vi "LineColorEnd.vi"(6 "Row":i32, 7 "Cluster":T1, 8 "error in":errorcluster, 9 "Event":bool, 11 "Result\n0.Item\n1.data\n2.limit\n3.result":string[](array[string])) -> (1 "SystemProcess":T2, 3 "Row":i32, 5 "output cluster":T1)   [LabVIEW 2013]
uses:
  Control/SystemProcess.ctl
  <vilib>/Utility/miscctls.llb/LVRowAndColumnTypeDef.ctl
  <vilib>/Utility/miscctls.llb/LVRowAndColumnUnsignedTypeDef.ctl
  Control/Read&Write.ctl
  Control/Buffer.vi
panel:
  out "Reserve:":string
  out "last":i32
  out "this":u32
  out "concatenated string":string
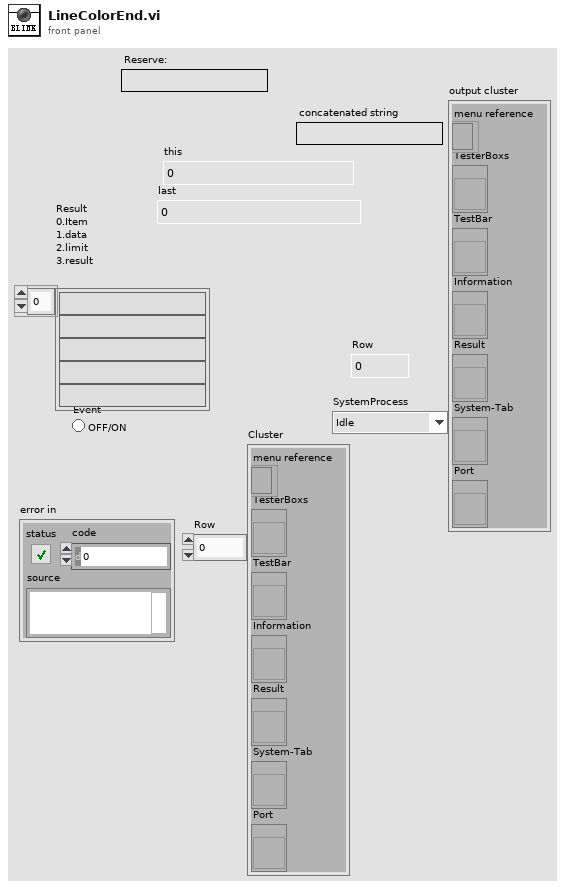
[diagram p1: front panel]
types:
  T1 = cluster{"menu reference":refnum<k9>, "TesterBoxs":refnum<vi>, "TestBar":refnum<vi>, "Information":refnum<vi>, "Result":refnum<vi>, "System-Tab":refnum<vi>, "Port":refnum<vi>}
  T2 = typedef "SystemProcess.ctl" = enum16{"Idle", "SystemInit", "SpecialEvent", "Barcode(SN)", "TestInitialize", "Test", "Stop", "SaveTestData", "Exit"}
  T3 = typedef "LVRowAndColumnUnsignedTypeDef.ctl" = cluster{"Row":u32, "Column":u32}
  T4 = typedef "LVRowAndColumnTypeDef.ctl" = cluster{"Row":i32, "Column":i32}
  T5 = typedef "Read&Write.ctl" = enum16{"Read", "Write"}
  T6 = typedef "StatusInformation.ctl" = cluster{"FileName:":string, "Barcode(S/N):":string, "TestStep:":string, "TestTime:":string, "Station:":string, "Model:":string, "Line:":string, "Status:":string, "Series:":string, "Reserve:":string}
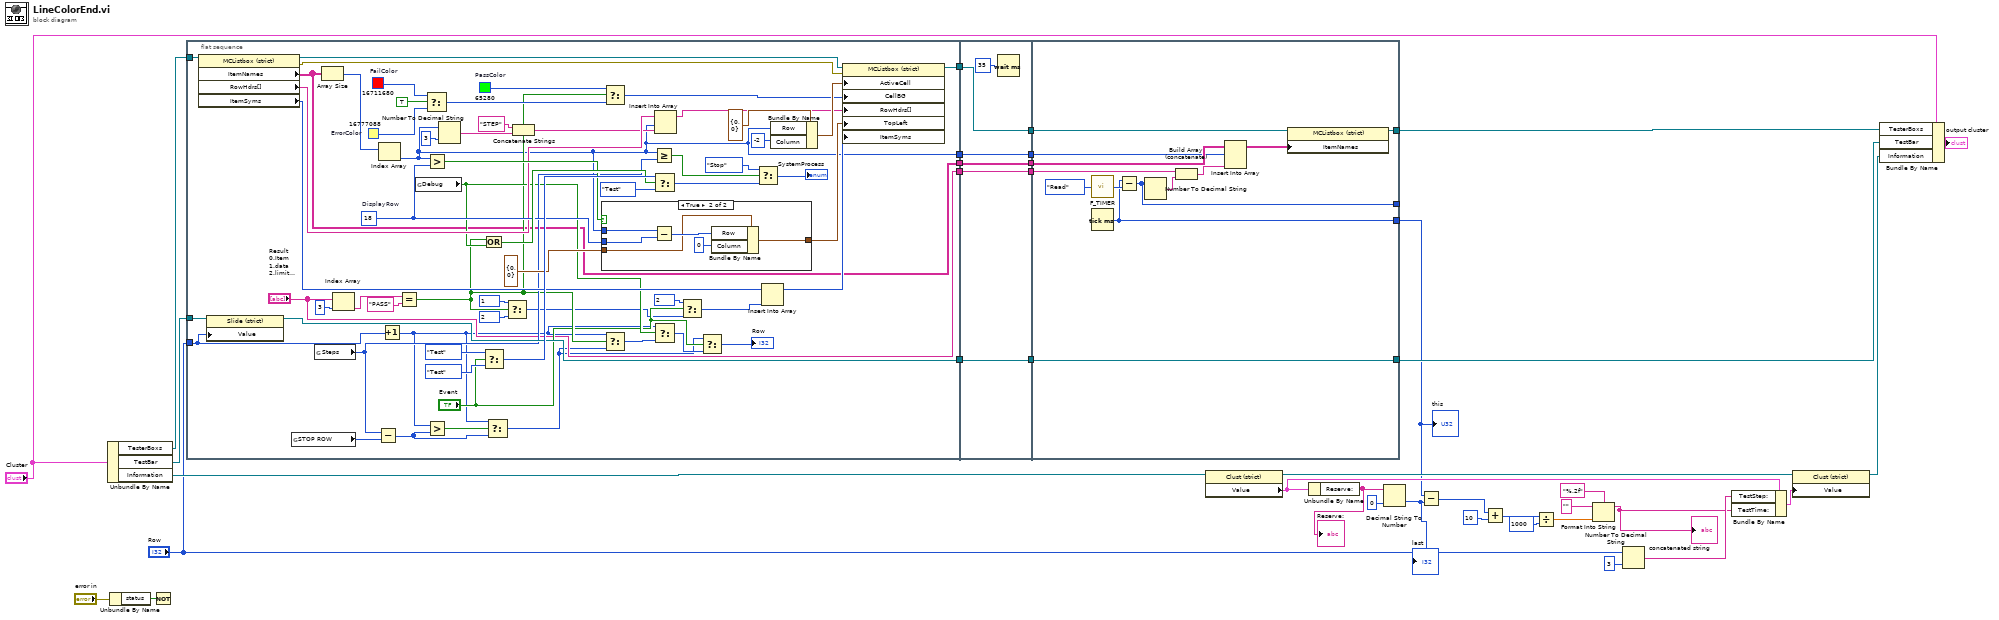
[diagram p0: block diagram]
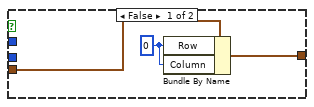
[diagram p2: hidden frame]
diagram:
  n1 = Unbundle By Name("Cluster") -> ("TesterBoxs"=w36:refnum<vi>, "TestBar"=w34:refnum<vi>, "Information"=w32:refnum<vi>)
  n2 = Unbundle By Name("error in") -> ("status"=w37:bool)
  n3 = Not(x=w37) -> ()  [unwired: 1 out]
  n4 = flat-sequence {
    tunnel: w36 -> [w67]
    tunnel: w34 -> [w65]
    tunnel: "Row" -> [w42]
    tunnel: [w66] -> w17
    tunnel: [w64] -> w15
    tunnel: [w46] -> w13
    tunnel: [w45] -> w11
    tunnel: ["Result\n0.Item\n1.data\n2.limit\n3.result"] -> w9
    tunnel: w17 -> [w114]
    tunnel: [w114] -> w16
    tunnel: w15 -> [w113]
    tunnel: [w113] -> w14
    tunnel: w13 -> [w112]
    tunnel: [w112] -> w12
    tunnel: w11 -> [w111]
    tunnel: [w111] -> w10
    tunnel: w9 -> [w110]
    tunnel: [w110] -> w8
    tunnel: [w127] -> w33
    tunnel: [w125] -> w35
    tunnel: [w116] -> w5
    tunnel: w8 -> [w119]
    tunnel: w10 -> [w122]
    tunnel: w12 -> [w123]
    tunnel: w14 -> [w127]
    tunnel: w16 -> [w126]
    tunnel: [w115] -> _
    frame #0 {
      w77 = 18  # DisplayRow
      w81 = u32 16777088  # ErrorColor
      w83 = u32 16711680  # FailColor
      w88 = u32 65280  # PassColor
      n5 = property class="MCListbox (strict)"(reference=w67) -> (reference out=w86:refnum<vi>, error out=w85:errorcluster, "ItemNames"=w46:string[][], "RowHdrs[]"=w73:string[], "ItemSyms"=w63:i32[])  [unwired: 1 in]
      n6 = property class="Slide (strict)"(reference=w65, "Value"=w42) -> (reference out=w64:refnum<vi>)  [unwired: 1 in, 1 out]
      n7 = global read "Buffer.vi" "STOP ROW"() -> (w47:i32)
      n8 = global read "Buffer.vi" "Steps"() -> (w59:i32)
      n9 = Array Size(array=w46) -> (size(s)=w84:i32[])
      n10 = Index Array(array="Result\n0.Item\n1.data\n2.limit\n3.result", index=3) -> (element=w93:string)
      n11 = Subtract(x=w59, y=w47) -> (x-y=w41:i32)
      n12 = Index Array(array=w84) -> (element=w45:i32)  [unwired: 1 in]
      n13 = Increment(x=w42) -> (x+1=w39:i32)
      n14 = Equal?(x=w93, y="PASS") -> (x = y?=w54:bool)
      n15 = global read "Buffer.vi" "Debug"() -> (w58:bool)
      n16 = Select(t=w83, s=TRUE, f=w81) -> (s? t:f=w82:u32)
      n17 = Greater?(x=w45, y=w77) -> (0:w78:bool)
      n18 = Greater?(x=w39, y=w41) -> (0:w43:bool)
      n19 = Number To Decimal String(number=w45, width (-)=i16 3) -> (decimal integer string=w69:string)
      n20 = Or(x=w54, y=w58) -> (x .or. y?=w80:bool)
      n21 = Select(t=SystemProcess."Test", s="Event", f=SystemProcess."Test") -> (s? t:f=w96:T2)
      n22 = Select(t=w39, s=w43, f=w41) -> (s? t:f=w40:i32)
      n23 = Select(t=1, s=w54, f=2) -> (s? t:f=w49:i32)
      n24 = Concatenate Strings("STEP" ("string"), w69) -> (w70:string)
      n25 = case shown="True" w78 {
        tunnel: w45 -> [_ w107]
        tunnel: [w102 w105] -> w75
        tunnel: w77 -> [_ w104]
        tunnel: T3 {"Row"=0, "Column"=0} ("Top Left Visible Cell") -> [w100 w103]
        frame False {
          w101 = u32 0 ("Column")
          n26 = Bundle By Name(cluster=w100, "Row"=w101, "Column"=w101) -> (w102:T3)
        }
        frame True {
          n27 = Subtract(x=w107, y=w104) -> (x-y=w106:i32)
          n28 = Bundle By Name(cluster=w103, "Row"=w106, "Column"=u32 0) -> (w105:T3)
        }
      }
      n29 = Select(t=w88, s=w54, f=w82) -> (s? t:f=w87:u32)
      n30 = Select(t=w39, s=w54, f=w40) -> (s? t:f=w57:i32)
      n31 = Greater Or Equal?(x=w45, y=w59) -> (x >= y?=w95:bool)
      n32 = Select(t=w96, s=w80, f=SystemProcess."Test") -> (s? t:f=w56:T2)
      n33 = Select(t=w39, s=w58, f=w57) -> (s? t:f=w53:i32)
      n34 = Insert Into Array(array=w73, index=w45, new element=w70) -> (w72:string[])
      n35 = Select(t=2, s="Event", f=w49) -> (s? t:f=w48:i32)
      n36 = Select(t=w40, s="Event", f=w53) -> (s? t:f=→"Row":i32)
      n37 = Select(t=SystemProcess."Stop" ("SystemProcess"), s=w95, f=w56) -> (s? t:f=→"SystemProcess":T2)
      n38 = Insert Into Array(array=w63, new element=w48) -> (w60:i32[])  [unwired: 1 in]
      n39 = Bundle By Name(cluster=T4 {"Row"=0, "Column"=0} ("Active Cell:Active Cell"), "Row"=w45, "Column"=-2) -> (w89:T4)
      n40 = property on="Property Node" class="MCListbox (strict)"(reference=w86, error in=w85, "ActiveCell"=w89, "CellBG"=w87, "RowHdrs[]"=w72, "TopLeft"=w75, "ItemSyms"=w60) -> (reference out=w66:refnum<vi>)  [unwired: 1 out]
    }
    frame #1 {
      n41 = Wait (ms)(milliseconds to wait=u32 35) -> ()  [unwired: 1 out]
    }
    frame #2 {
      n42 = call "F_TIMER.vi"("Enum-Read/Write"=Read&Write."Read") -> ("timer"=w121:u32)
      n43 = Tick Count (ms)() -> (millisecond timer value=w116:u32)
      n44 = Subtract(x=w116, y=w121) -> (x-y=w115:u32)
      n45 = Number To Decimal String(number=w115) -> (decimal integer string=w118:string)  [unwired: 1 in]
      n46 = Build Array (concatenate)(w119, w118) -> (w117:string[])
      n47 = Insert Into Array(array=w123, index (row)=w122, new element=w117) -> (w124:string[][])  [unwired: 1 in]
      n48 = property class="MCListbox (strict)"(reference=w126, "ItemNames"=w124) -> (reference out=w125:refnum<vi>)  [unwired: 1 in, 1 out]
    }
  }
  n49 = property class="Clust (strict)"(reference=w32) -> (reference out=w24:refnum<vi>, "Value"=w28:T6)  [unwired: 1 in, 1 out]
  n50 = Unbundle By Name(w28) -> ("Reserve:"=w31:string)
  "Reserve:" <- w31
  n51 = Decimal String To Number(string=w31, default (0L)=i64 0 ("default (0 I32)")) -> (number=w30:i64)  [unwired: 1 in, 1 out]
  "last" <- w30
  n52 = Subtract(x=w5, y=w30) -> (x-y=w2:i64)
  n53 = Add(x=w2, y=u32 10 ("Torlance")) -> (x+y=w18:i64)
  n54 = Divide(x=w18, y=u32 1000) -> (x/y=w21:dbl)
  n55 = Format Into String(format string="%.2f", initial string="", w21) -> (resulting string=w3:string)  [unwired: 1 in, 1 out]
  "concatenated string" <- w3
  n56 = Number To Decimal String(number="Row", width (-)=i16 3) -> (decimal integer string=w26:string)
  n57 = Bundle By Name(cluster=w28, "TestStep:"=w26, "TestTime:"=w3) -> (w23:T6)
  n58 = property class="Clust (strict)"(reference=w24, "Value"=w23) -> (reference out=w22:refnum<vi>)  [unwired: 1 in, 1 out]
  n59 = Bundle By Name(cluster="Cluster", "TesterBoxs"=w35, "TestBar"=w33, "Information"=w22) -> (→"output cluster":T1)
  "this" <- w5
